vi "SN处1理.vi"(7 "动作":enum16{"Check", "Regist"}(ring), 11 "SN号":i32=337645664) -> (3 "SN":u32)   [LabVIEW 2011]
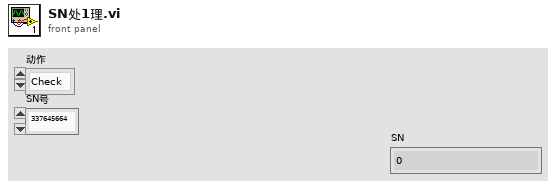
[diagram p1: front panel]
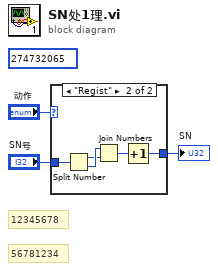
[diagram p0: block diagram]
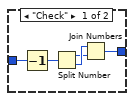
[diagram p2: hidden frame]
diagram:
  (unwired) 274732065
  # "56781234"
  # "12345678"
  n1 = case shown="\"Regist\"" "动作" {
    tunnel: "SN号" -> [w8 w13]
    tunnel: [w4 w9] -> w2
    frame "Check" {
      n2 = Decrement(x=w8) -> (x-1=w5:i32)
      n3 = Split Number(x=w5) -> (hi(x)=w6:u16, lo(x)=w7:u16)
      n4 = Join Numbers(hi=w7, lo=w6) -> ((hi.lo)=w4:u32)
    }
    frame "Regist" {
      n5 = Split Number(x=w13) -> (hi(x)=w11:u16, lo(x)=w12:u16)
      n6 = Join Numbers(hi=w12, lo=w11) -> ((hi.lo)=w10:u32)
      n7 = Increment(x=w10) -> (x+1=w9:u32)
    }
  }
  "SN" <- w2
